vi "Create Test Report from Template.vi"() -> ()   [LabVIEW 2013]
panel:
  in  "Add to Project":u16(ring) items=["<no project selected>", "Caraya.lvproj"]
  in  "Create Test Report Class":bool
  in  "Destination Folder":path
  in  "New Test Report Class Name":string
  # "CARAYA Custom Test Report Class Creator\n\nFill in the destination folder and new TestReport class name."
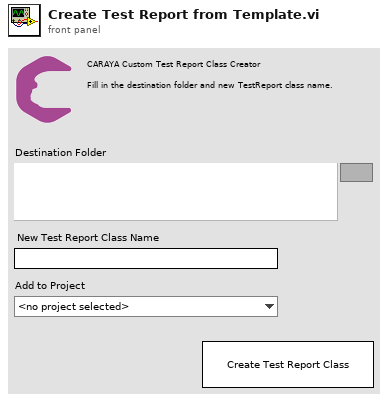
[diagram p1: front panel]
types:
  T1 = enum32{"invalid app kind", "Development System", "Run Time System", "Student Edition", "Embedded LabVIEW", "Evaluation", "Custom"}
  T2 = enum8{"Enabled", "Disabled", "Disabled and Grayed Out"}
  T3 = enum32{"Invalid", "Standard", "Closed", "Hidden", "Minimized", "Maximized"}
  T4 = cluster{"Core":cluster{"Current VI Reference":refnum<vi>, "Close Panel on Exit?":bool}, "ClassName":string, "Path":path, "auto-path":bool, "Menu Launch AppRef":refnum<vi>, "Projects[]":refnum<vi>[], "NewClassPath":path}
  T5 = cluster{"Current VI Reference":refnum<vi>, "Close Panel on Exit?":bool}
  T6 = enum32{"Invalid", "Standard", "Closed", "Hidden", "Minimized", "Maximized"}[]
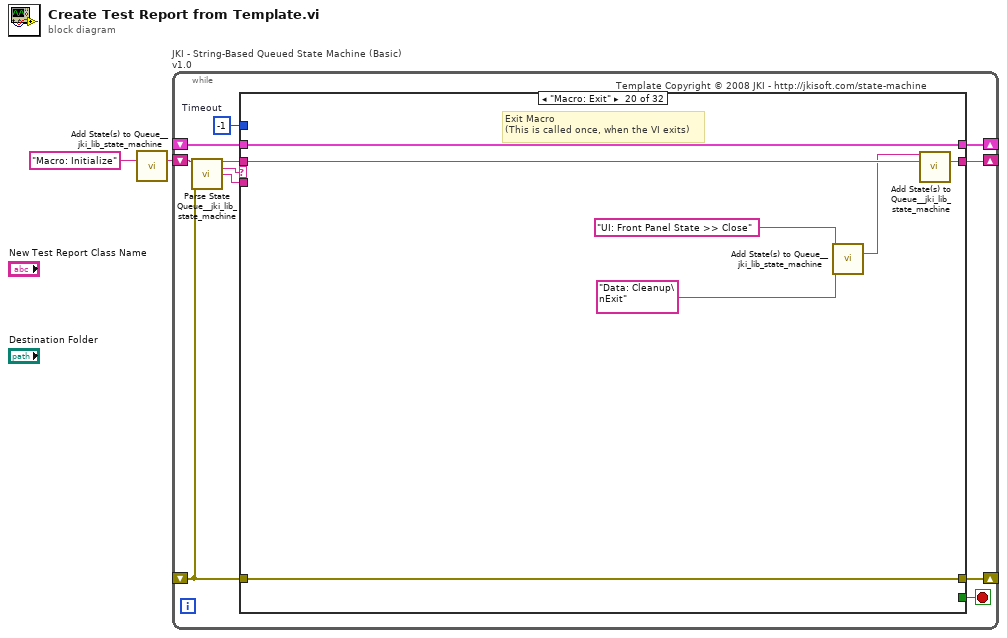
[diagram p0: block diagram]
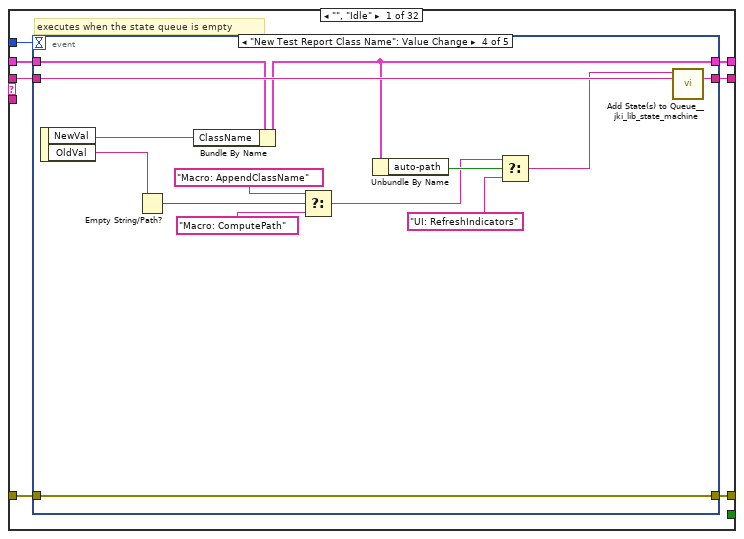
[diagram p2: hidden frame]
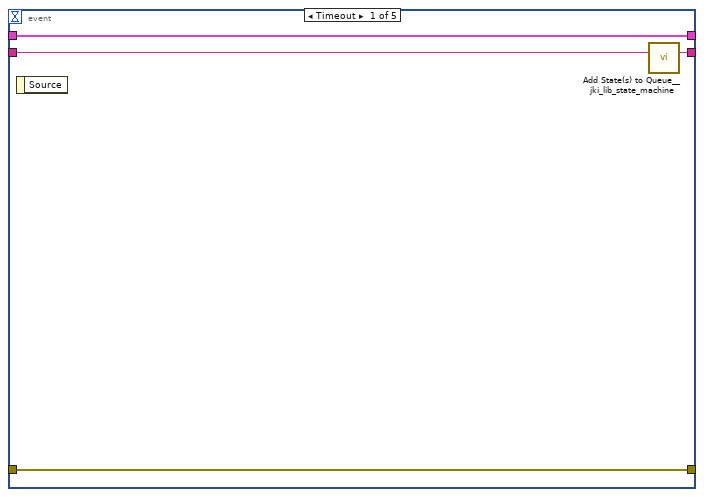
[diagram p3: hidden frame]
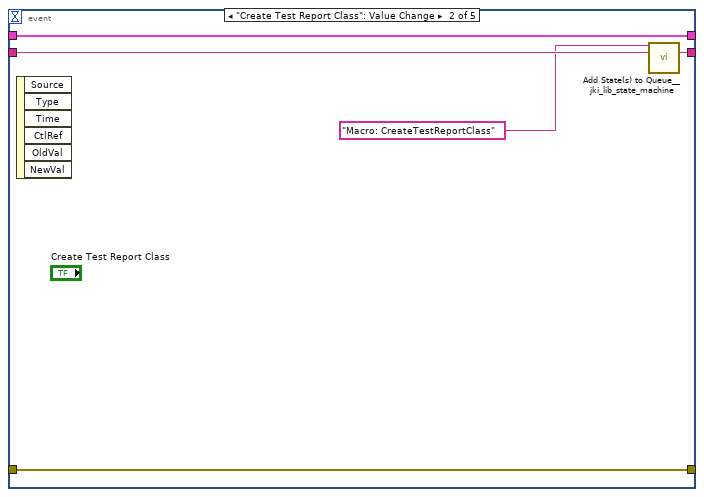
[diagram p4: hidden frame]
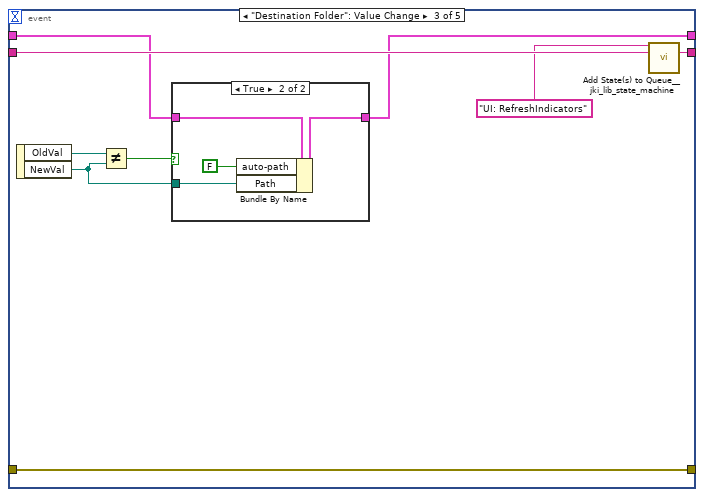
[diagram p5: hidden frame]
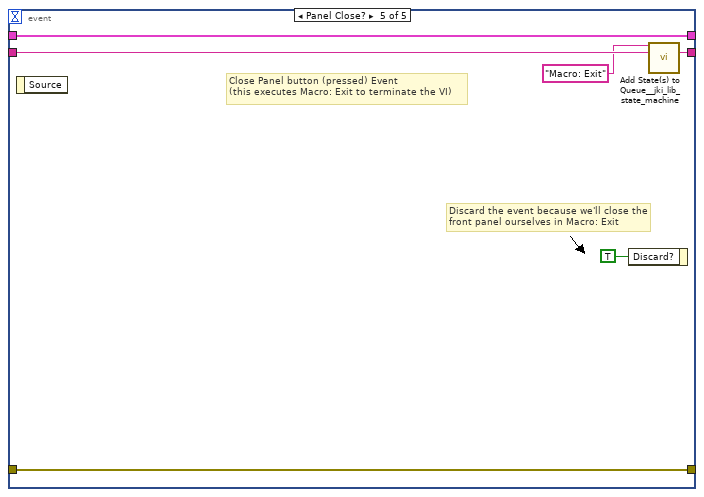
[diagram p7: hidden frame]
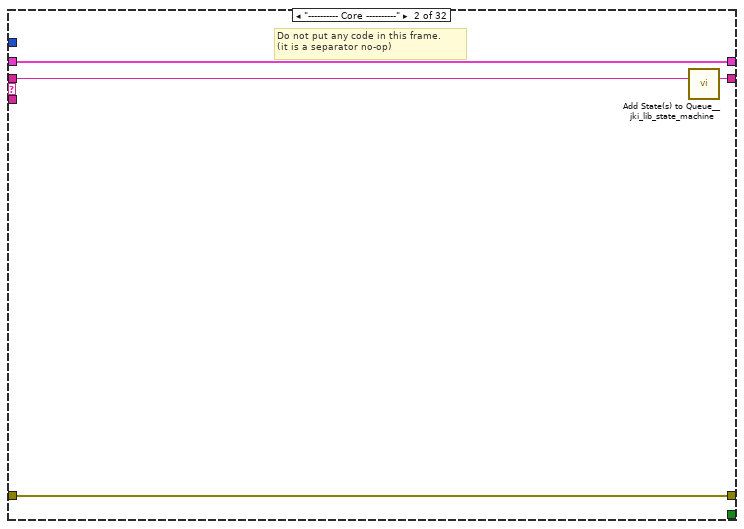
[diagram p8: hidden frame]
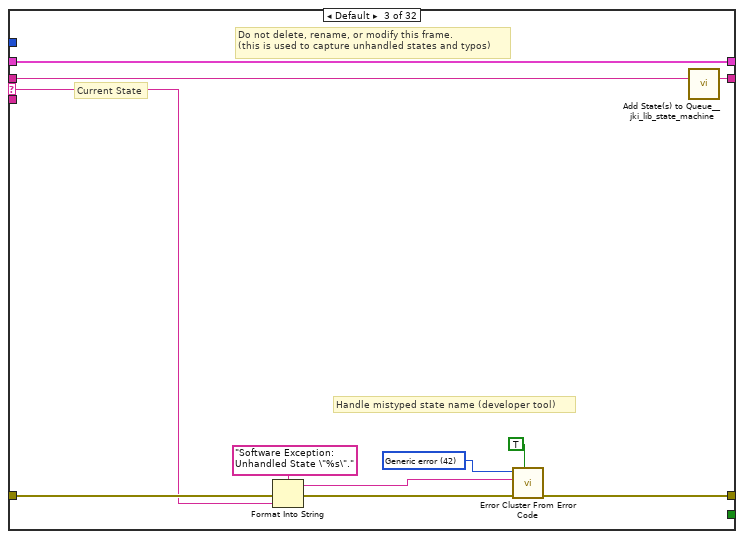
[diagram p9: hidden frame]
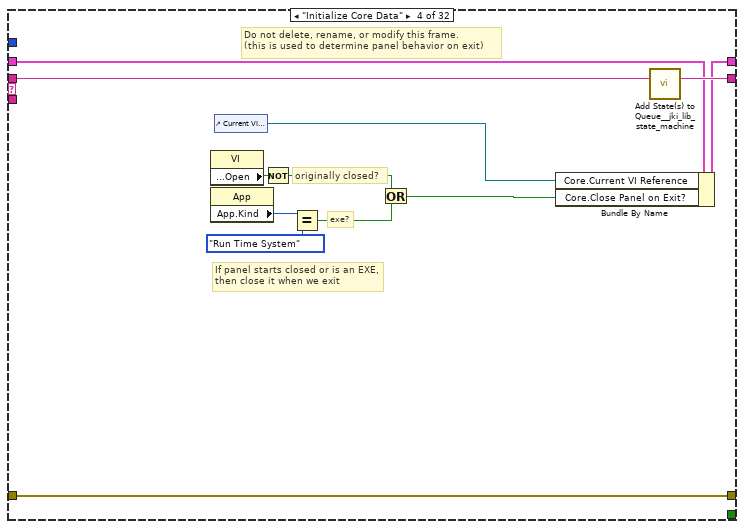
[diagram p10: hidden frame]
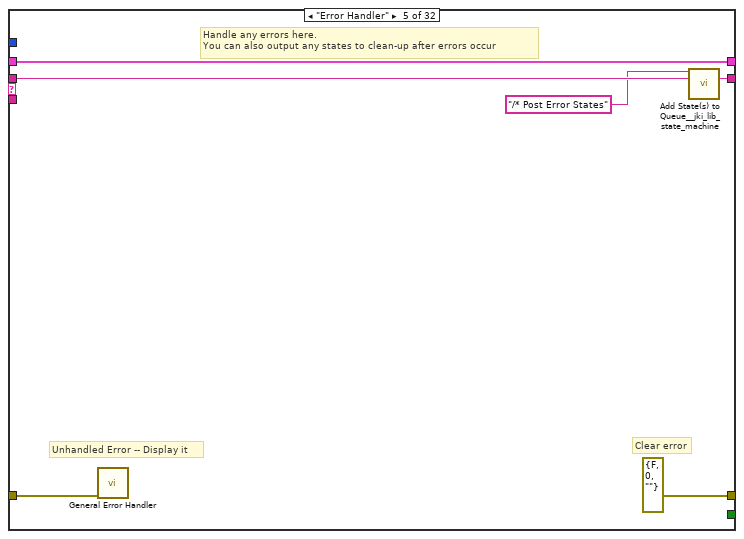
[diagram p11: hidden frame]
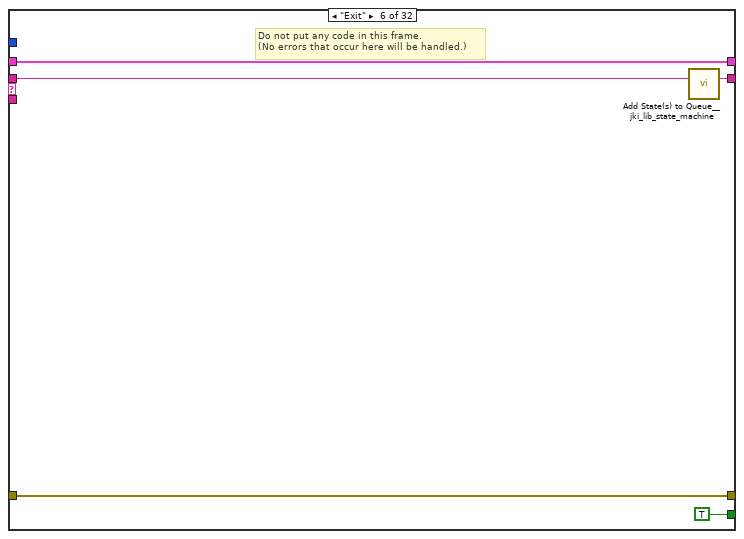
[diagram p12: hidden frame]
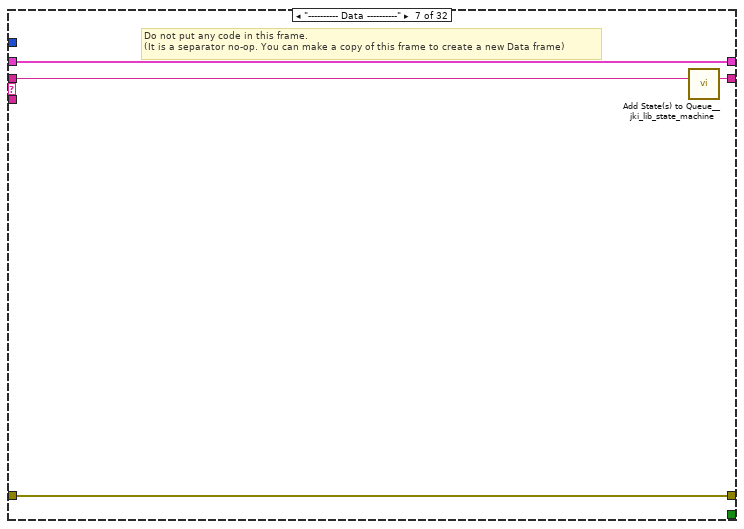
[diagram p13: hidden frame]
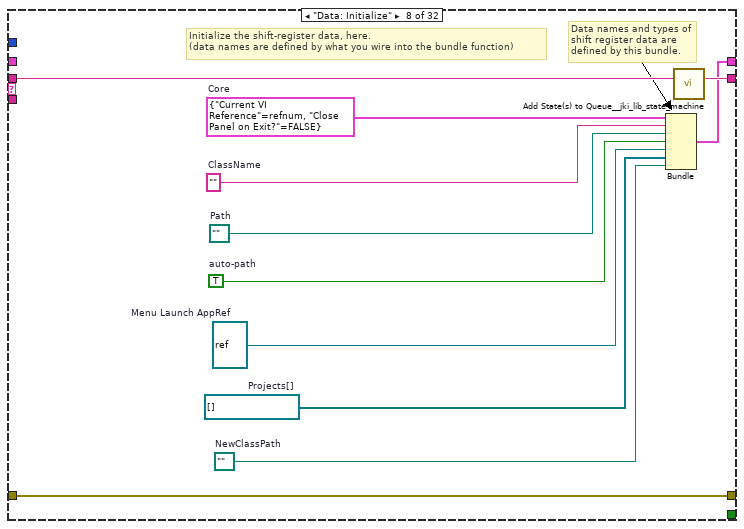
[diagram p14: hidden frame]
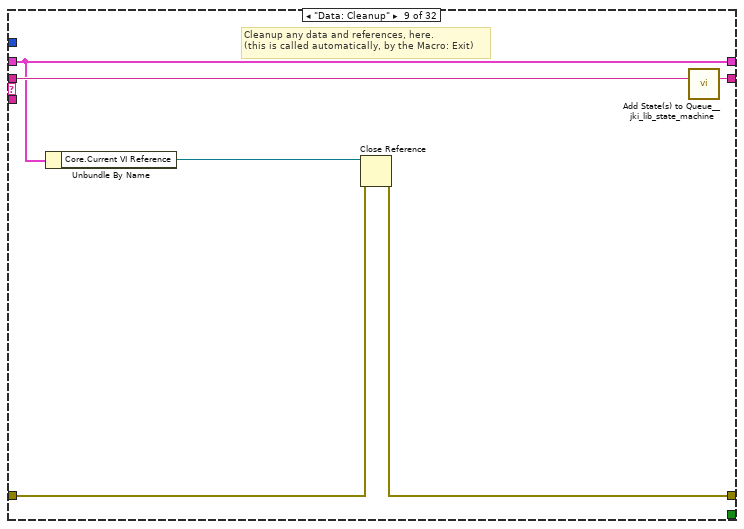
[diagram p15: hidden frame]
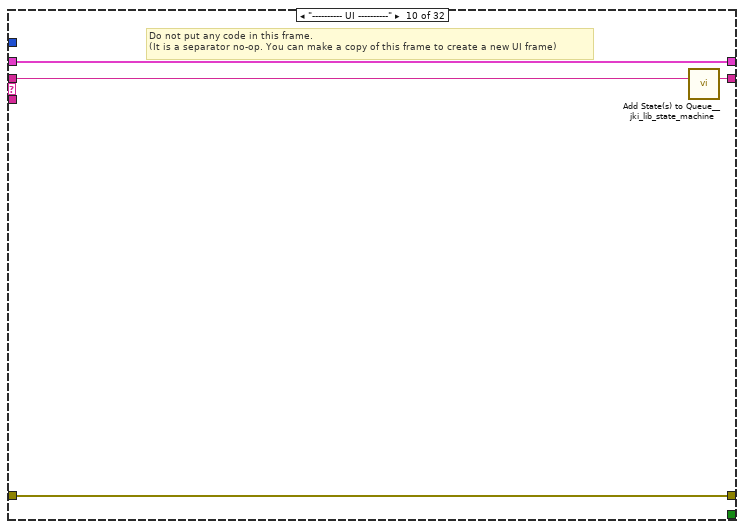
[diagram p16: hidden frame]
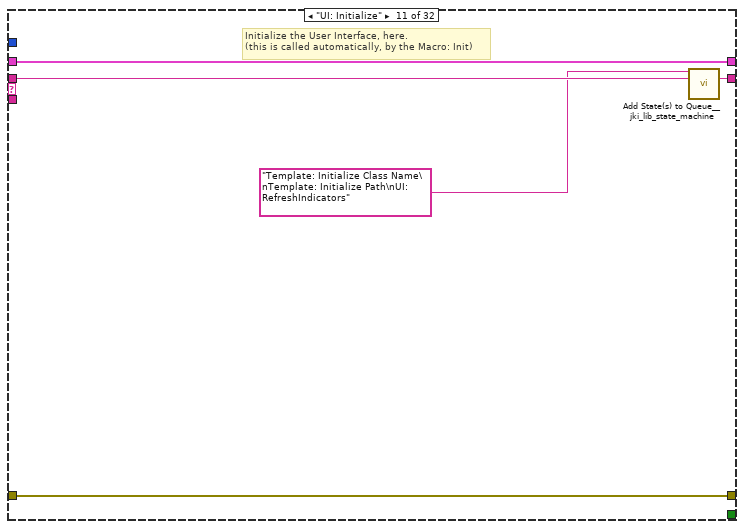
[diagram p17: hidden frame]
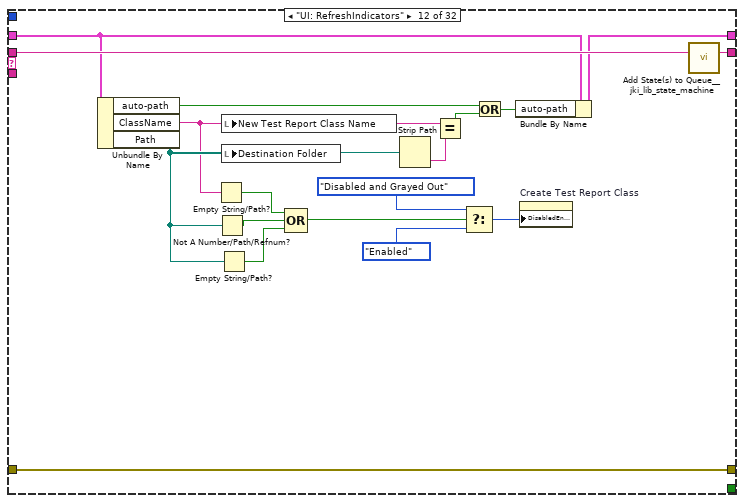
[diagram p18: hidden frame]
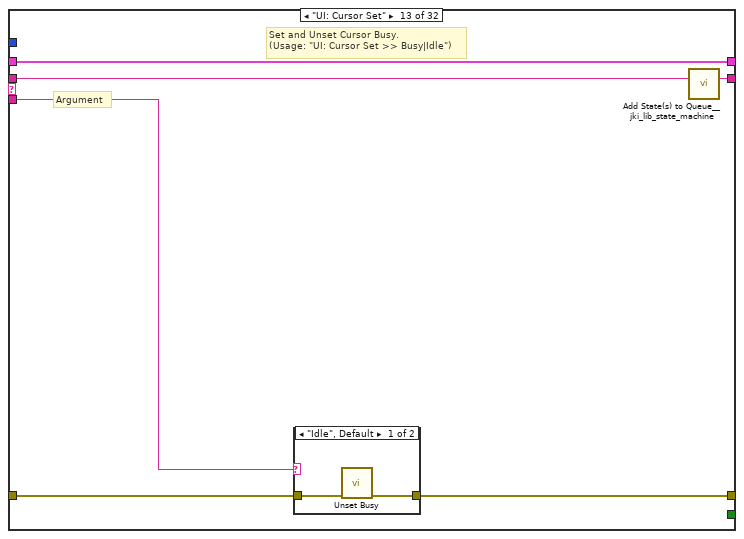
[diagram p19: hidden frame]
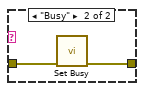
[diagram p20: hidden frame]
diagram:
  n1 = call <vilib>:"Add State(s) to Queue__jki_lib_state_machine.vi"("State(s) in (\"\")"="Macro: Initialize") -> ("States Out"=w2:string)  [unwired: 14 in]
  n2 = while "JKI - String-Based Queued State Machine (Basic) v1.0" {
    shift-right: [w6] -> _
    shift-left: _ -> [w5]
    shift-right: [w9] -> _
    shift-left: _ -> [w3]
    shift-right: [w8] -> _
    shift-left: w2 -> [w10]
    stop <- w7 stop-if-true
    w4 = -1  # Timeout
    # "Template Copyright © 2008 JKI - http://jkisoft.com/state-machine"
    n3 = call <vilib>:"Parse State Queue__jki_lib_state_machine.vi"("State Queue"=w10, "Error In (no error)"=w3) -> ("Remaining States"=w12:string, "Current State"=w13:string, "Arguments"=w11:string)  [unwired: 11 in]
    n4 = case shown="\"Macro: Exit\"" w13 {
      selector: w13 -> [_ _ w68 _ _ _ _ _ _ _ _ _ _ _ _ _ _ _ _ _ _ _ _ _ _ _ _ _ _ _ _ _]
      tunnel: w12 -> [w20 w67 w72 w90 w96 w101 w105 w116 w122 w126 w131 w149 w155 w166 w192 w197 w202 w207 w212 w219 w223 w238 w246 w254 w270 w299 w320 w349 w359 w369 w379 w389]
      tunnel: w11 -> [_ _ _ _ _ _ _ _ _ _ _ _ w150 w160 _ _ _ _ _ _ _ _ _ _ _ _ _ _ _ _ _ _]
      tunnel: w5 -> [w18 w64 w70 w81 w93 w99 w102 _ w117 w123 w128 w136 w153 w162 w189 w194 w199 w204 w209 w216 w220 w236 w243 w248 w259 w295 w316 w345 w354 w364 w374 w387]
      tunnel: [w17 w65 w74 w87 errorcluster {"status"=FALSE, "code"=0, "source"=""} ("error out") w98 w103 w113 w118 w124 w129 w147 w151 w163 w190 w195 w200 w205 w210 w217 w221 w224 w244 w252 w268 w297 w318 w332 w350 w360 w370 w380] -> w9
      tunnel: w3 -> [w16 w65 w73 w87 w92 w98 w103 w113 w119 w124 w129 w147 w152 w164 w190 w195 w200 w205 w210 w217 w221 w225 w244 w252 w268 w297 w318 w335 w356 w366 w376 w381]
      tunnel: [w19 w66 w71 w89 w95 w100 w104 w115 w121 w125 w130 w148 w154 w165 w191 w196 w201 w206 w211 w218 w222 w237 w245 w253 w269 w298 w319 w348 w358 w368 w378 w388] -> w8
      tunnel: [_ _ _ _ _ TRUE _ _ _ _ _ _ _ _ _ _ _ _ _ _ _ _ _ _ _ _ _ _ _ _ _ _] -> w7
      tunnel: [w15 w64 w70 w88 w93 w99 w102 w114 w117 w123 w128 w135 w153 w162 w189 w194 w199 w204 w209 w216 w220 w235 w243 w247 w267 w296 w317 w344 w354 w364 w374 w387] -> w6
      tunnel: w4 -> [w14 _ _ _ _ _ _ _ _ _ _ _ _ _ _ _ _ _ _ _ _ _ _ _ _ _ _ _ _ _ _ _]
      frame "", "Idle" {
        # "executes when the state queue is empty"
        n5 = event shown="[3] \"New Test Report Class Name\": Value Change" {
          selector: _ -> [_ _ _ _ _]
          dyn-events: _ -> [_ _ _ _ _]
          timeout: w14 -> [_ _ _ _ _]
          tunnel: w20 -> [w24 w29 w38 w57 w63]
          tunnel: [w23 w28 w37 w56 w62] -> w19
          tunnel: w18 -> [w21 w26 w34 w54 w60]
          tunnel: [w22 w27 w36 w55 w61] -> w17
          tunnel: w16 -> [w22 w27 w36 w55 w61]
          tunnel: [w21 w26 w31 w53 w60] -> w15
          event Timeout {
            n6 = event-data() -> ()  [unwired: 1 in, 1 out]
            n7 = call <vilib>:"Add State(s) to Queue__jki_lib_state_machine.vi"("State(s) in (\"\")"=w24) -> ("States Out"=w23:string)  [unwired: 14 in]
          }
          event "Create Test Report Class": Value Change {
            n8 = event-data() -> ()  [unwired: 1 in, 6 out]
            n9 = call <vilib>:"Add State(s) to Queue__jki_lib_state_machine.vi"("State(s) in Front (\"\")"="Macro: CreateTestReportClass", "State(s) in (\"\")"=w29) -> ("States Out"=w28:string)  [unwired: 13 in]
          }
          event "Destination Folder": Value Change {
            n10 = event-data() -> ("OldVal"=w35:path, "NewVal"=w32:path)  [unwired: 1 in]
            n11 = Not Equal?(x=w35, y=w32) -> (x != y?=w33:bool)
            n12 = case shown="True" w33 {
              tunnel: [w39 w43] -> w31
              tunnel: w34 -> [w39 w42]
              tunnel: w32 -> [_ w41]
              frame False {
              }
              frame True {
                n13 = Bundle By Name(cluster=w42, "auto-path"=FALSE, "Path"=w41) -> (w43:T4)
              }
            }
            n14 = call <vilib>:"Add State(s) to Queue__jki_lib_state_machine.vi"("State(s) in Front (\"\")"="UI: RefreshIndicators", "State(s) in (\"\")"=w38) -> ("States Out"=w37:string)  [unwired: 13 in]
          }
          event "New Test Report Class Name": Value Change {
            n15 = event-data() -> ("NewVal"=w52:string, "OldVal"=w49:string)  [unwired: 1 in]
            n16 = Empty String/Path?(string/path=w49) -> (empty?=w48:bool)
            n17 = Bundle By Name(cluster=w54, "ClassName"=w52) -> (w53:T4)
            n18 = Select(t="Macro: AppendClassName", s=w48, f="Macro: ComputePath") -> (s? t:f=w45:string)
            n19 = Unbundle By Name(w53) -> ("auto-path"=w51:bool)
            n20 = Select(t=w45, s=w51, f="UI: RefreshIndicators") -> (s? t:f=w50:string)
            n21 = call <vilib>:"Add State(s) to Queue__jki_lib_state_machine.vi"("State(s) in Front (\"\")"=w50, "State(s) in (\"\")"=w57) -> ("States Out"=w56:string)  [unwired: 13 in]
          }
          event Panel Close? {
            # "Discard the event because we'll close the front panel ourselves in Macro: Exit"
            # "Close Panel button (pressed) Event\n(this executes Macro: Exit to terminate the VI)"
            n22 = event-data() -> ()  [unwired: 1 in, 1 out]
            n23 = event-data("Discard?"=TRUE) -> ()  [unwired: 1 in, 1 out]
            n24 = call <vilib>:"Add State(s) to Queue__jki_lib_state_machine.vi"("State(s) in Front (\"\")"="Macro: Exit", "State(s) in (\"\")"=w63) -> ("States Out"=w62:string)  [unwired: 13 in]
          }
        }
      }
      frame "---------- Core ----------" {
        # "Do not put any code in this frame.\n(it is a separator no-op)"
        n25 = call <vilib>:"Add State(s) to Queue__jki_lib_state_machine.vi"("State(s) in (\"\")"=w67) -> ("States Out"=w66:string)  [unwired: 14 in]
      }
      frame Default {
        w77 = 42 items=["No error", "Argument error", "Memory is full", "Out of zone", "End of file", "File already open", "Generic file I/O error", "File not found", "File permission error", "Disk is full", "Duplicate path", "Too many files open", "System feature not enabled", "Resource file not found", "Cannot add resource", "Resource not found", "Image not found", "Image memory error", "Pen does not exist", "Config type invalid", "Config token not found", "Config parse error", "Config memory error", "Bad external code format", "Bad external code offset", "External code not present", "Null window", "Destroy window error", "Null menu", "Print aborted", "Bad print record", "Print driver error", "Windows error during printing", "Memory error during printing", "Print dialog error", "Generic print error", "Invalid device refnum", "Device not found", "Device parameter error", "Device unit error", "Cannot open device", "Device call aborted", "Generic error", "Cancelled by user", "Object ID too low", "Object ID too high", "Object not in heap", "Unknown heap", "Unknown object (invalid DefProc)", "Unknown object (DefProc not in table)", "Message out of range", "Invalid (null) method", "Unknown message", "Manager call not supported", "Bad address", "Network operation in progress", "Network operation timed out", "Connection is busy", "Network attribute not supported", "Network error", "Address in use", "System out of memory", "Connection aborted", "Connection refused", "Not connected", "Already connected", "Connection closed", "Initialization error (interapplication manager)", "Bad occurrence", "Wait on unbound occurrence handler", "Occurrence queue overflow", "Datalog type conflict", "Unused", "Unrecognized type (interapplication manager)", "Memory corrupt", "Failed to make temporary DLL", "Old CIN version", "Drag socket not found", "Failed to load drop-object", "Failed to register OLE object", "Failed to release OLE object", "Format specifier type mismatch", "Unknown format specifier", "Too few format specifiers", "Too many format specifiers", "Scan failed", "Newer CIN version", "Error converting to variant", "Runtime menu error", "Password tampered", "Variant attribute not found", "Incompatible variant data type", "Event data is not available", "Event Store is not present", "Occurrence is not found", "Event Queue is not created", "Event info is not available", "Refnum passed is NULL", "Error retrieving Class GUID", "Error retrieving CoClass GUID", "Error retrieving TypeLib GUID.", "Bad built application magic bytes.", "Specific driver is different from the specific driver associated with the Logical Name.", "There is no session opened to the class driver.", "Max Error", "MAX - Error with config objects", "MAX - Error loading configuration", "MAX - Group not supported"]
        # "Current State"
        # "Do not delete, rename, or modify this frame.\n(this is used to capture unhandled states and typos)"
        # "Handle mistyped state name (developer tool)"
        n26 = Format Into String(format string="Software Exception: Unhandled State \"%s\"." ("message"), error in=w73, w68) -> (resulting string=w76:string, error out=w75:errorcluster)  [unwired: 1 in]
        n27 = call <vilib>:"Error Cluster From Error Code.vi"("show call chain? (False)"=TRUE, "error in (no error)"=w75, "error message (\"\")"=w76, "error code (0)"=w77) -> ("error out"=w74:errorcluster)  [unwired: 5 in]
        n28 = call <vilib>:"Add State(s) to Queue__jki_lib_state_machine.vi"("State(s) in (\"\")"=w72) -> ("States Out"=w71:string)  [unwired: 14 in]
      }
      frame "Initialize Core Data" {
        # "Do not delete, rename, or modify this frame.\n(this is used to determine panel behavior on exit)"
        # "originally closed?"
        # "exe?"
        # "If panel starts closed or is an EXE, then close it when we exit"
        n29 = property class="VI"() -> ("Front Panel.Open"=w86:bool)  [unwired: 2 in, 2 out]
        n30 = property class="App"() -> ("App.Kind"=w85:T1)  [unwired: 2 in, 2 out]
        n31 = control-ref of="Current VI Reference"() -> (w79:refnum<vi>)
        n32 = Not(x=w86) -> (.not. x?=w83:bool)
        n33 = Equal?(x=w85, y=T1."Run Time System" ("Application:Kind")) -> (x = y?=w82:bool)
        n34 = Or(x=w83, y=w82) -> (x .or. y?=w80:bool)
        n35 = Bundle By Name(cluster=w81, "Core.Current VI Reference"=w79, "Core.Close Panel on Exit?"=w80) -> (w88:T4)
        n36 = call <vilib>:"Add State(s) to Queue__jki_lib_state_machine.vi"("State(s) in (\"\")"=w90) -> ("States Out"=w89:string)  [unwired: 14 in]
      }
      frame "Error Handler" {
        # "Unhandled Error -- Display it"
        # "Handle any errors here.\nYou can also output any states to clean-up after errors occur"
        # "Clear error"
        n37 = call <vilib>:"General Error Handler.vi"("error in (no error)"=w92) -> ()  [unwired: 10 in, 5 out]
        n38 = call <vilib>:"Add State(s) to Queue__jki_lib_state_machine.vi"("State(s) in Front (\"\")"="/* Post Error States", "State(s) in (\"\")"=w96) -> ("States Out"=w95:string)  [unwired: 13 in]
      }
      frame "Exit" {
        # "Do not put any code in this frame.\n(No errors that occur here will be handled.)"
        n39 = call <vilib>:"Add State(s) to Queue__jki_lib_state_machine.vi"("State(s) in (\"\")"=w101) -> ("States Out"=w100:string)  [unwired: 14 in]
      }
      frame "---------- Data ----------" {
        # "Do not put any code in this frame.\n(It is a separator no-op. You can make a copy of this frame to create a new Data frame)"
        n40 = call <vilib>:"Add State(s) to Queue__jki_lib_state_machine.vi"("State(s) in (\"\")"=w105) -> ("States Out"=w104:string)  [unwired: 14 in]
      }
      frame "Data: Initialize" {
        w106 = path ""  # NewClassPath
        w107 = refnum<vi>[] []  # Projects[]
        w108 = refnum<vi> refnum  # Menu Launch AppRef
        w109 = TRUE  # auto-path
        w110 = path ""  # Path
        w111 = T5 {"Current VI Reference"=refnum, "Close Panel on Exit?"=FALSE}  # Core
        w112 = ""  # ClassName
        # "Data names and types of shift register data are defined by this bundle."
        # "Initialize the shift-register data, here.\n(data names are defined by what you wire into the bundle function)"
        n41 = Bundle("Core"=w111, "ClassName"=w112, "Path"=w110, "auto-path"=w109, "Menu Launch AppRef"=w108, "Projects[]"=w107, "NewClassPath"=w106) -> (w114:T4)  [unwired: 1 in]
        n42 = call <vilib>:"Add State(s) to Queue__jki_lib_state_machine.vi"("State(s) in (\"\")"=w116) -> ("States Out"=w115:string)  [unwired: 14 in]
      }
      frame "Data: Cleanup" {
        # "Cleanup any data and references, here.\n(this is called automatically, by the Macro: Exit)"
        n43 = Unbundle By Name(w117) -> ("Core.Current VI Reference"=w120:refnum<vi>)
        n44 = Close Reference(reference=w120, error in (no error)=w119) -> (error out=w118:errorcluster)
        n45 = call <vilib>:"Add State(s) to Queue__jki_lib_state_machine.vi"("State(s) in (\"\")"=w122) -> ("States Out"=w121:string)  [unwired: 14 in]
      }
      frame "---------- UI ----------" {
        # "Do not put any code in this frame.\n(It is a separator no-op. You can make a copy of this frame to create a new UI frame)"
        n46 = call <vilib>:"Add State(s) to Queue__jki_lib_state_machine.vi"("State(s) in (\"\")"=w126) -> ("States Out"=w125:string)  [unwired: 14 in]
      }
      frame "UI: Initialize" {
        # "Initialize the User Interface, here.\n(this is called automatically, by the Macro: Init)"
        n47 = call <vilib>:"Add State(s) to Queue__jki_lib_state_machine.vi"("State(s) in Front (\"\")"="Template: Initialize Class Name\nTemplate: Initialize Path\nUI: RefreshIndicators" ("Text.Text"), "State(s) in (\"\")"=w131) -> ("States Out"=w130:string)  [unwired: 13 in]
      }
      frame "UI: RefreshIndicators" {
        n48 = Unbundle By Name(w136) -> ("auto-path"=w134:bool, "ClassName"=w137:string, "Path"=w139:path)
        n49 = Empty String/Path?(string/path=w137) -> (empty?=w146:bool)
        n50 = Not A Number/Path/Refnum?(number/path/refnum=w139) -> (NaN/Path/Refnum?=w145:bool)
        n51 = Empty String/Path?(string/path=w139) -> (empty?=w144:bool)
        n52 = local write "New Test Report Class Name"(w137) -> ()
        n53 = local write "Destination Folder"(w139) -> ()
        n54 = Compound Arithmetic op=OR(w146, w145, w144) -> (w142:bool)
        n55 = Strip Path(path=w139) -> (name=w138:string)  [unwired: 1 out]
        n56 = Equal?(x=w137, y=w138) -> (x = y?=w133:bool)
        n57 = Select(t=T2."Disabled and Grayed Out" ("Disabled"), s=w142, f=T2."Enabled" ("Disabled")) -> (s? t:f=w140:T2)
        n58 = Or(x=w134, y=w133) -> (x .or. y?=w132:bool)
        n59 = Bundle By Name(cluster=w136, "auto-path"=w132) -> (w135:T4)
        n60 = property on="Create Test Report Class" class="Bool"("DisabledEnum"=w140) -> ()  [unwired: 2 in, 2 out]
        n61 = call <vilib>:"Add State(s) to Queue__jki_lib_state_machine.vi"("State(s) in (\"\")"=w149) -> ("States Out"=w148:string)  [unwired: 14 in]
      }
      frame "UI: Cursor Set" {
        # "Argument"
        # "Set and Unset Cursor Busy.\n(Usage: \"UI: Cursor Set >> Busy|Idle\")"
        n62 = case shown="\"Idle\", Default" w150 {
          tunnel: w152 -> [w157 w159]
          tunnel: [w156 w158] -> w151
          frame "Idle", Default {
            n63 = call <vilib>:"Unset Busy.vi"("error in (no error)"=w157) -> ("error out"=w156:errorcluster)  [unwired: 10 in]
          }
          frame "Busy" {
            n64 = call <vilib>:"Set Busy.vi"("error in (no error)"=w159) -> ("error out"=w158:errorcluster)  [unwired: 9 in, 1 out]
          }
        }
        n65 = call <vilib>:"Add State(s) to Queue__jki_lib_state_machine.vi"("State(s) in (\"\")"=w155) -> ("States Out"=w154:string)  [unwired: 14 in]
      }
      frame "UI: Front Panel State" {
        # "Argument"
        # "Set Front Panel Open or Closed\n(Usage: \"UI: Front Panel State >> Open|Close\")"
        n66 = Unbundle By Name(w162) -> ("Core.Current VI Reference"=w161:refnum<vi>)
        n67 = case shown="\"Open\", Default" w160 {
          tunnel: w164 -> [w170 w183]
          tunnel: [w172 w184] -> w163
          tunnel: w161 -> [w171 w181]
          frame "Open", Default {
            n68 = property class="VI"(reference=w171, error in=w170) -> (reference out=w168:refnum<vi>, error out=w169:errorcluster, "Front Panel.Open"=w167:bool)
            n69 = case shown="False" w167 {
              tunnel: [w175 w178] -> w172
              tunnel: w169 -> [w174 w178]
              tunnel: w168 -> [w173 _]
              frame False {
                n70 = invoke class="VI" method="FP.Open"(reference=w173, error in=w174, "Activate"=TRUE, "State"=T3."Standard") -> (error out=w175:errorcluster)  [unwired: 1 in, 4 out]
              }
              frame True {
              }
            }
          }
          frame "Close" {
            n71 = property class="VI"(reference=w181, error in=w183) -> (reference out=w180:refnum<vi>, error out=w182:errorcluster, "Front Panel.Open"=w179:bool)
            n72 = case shown="True" w179 {
              tunnel: [w185 w188] -> w184
              tunnel: w182 -> [w185 w187]
              tunnel: w180 -> [_ w186]
              frame False {
              }
              frame True {
                n73 = invoke class="VI" method="FP.Close"(reference=w186, error in=w187) -> (error out=w188:errorcluster)  [unwired: 1 in, 2 out]
              }
            }
          }
        }
        n74 = call <vilib>:"Add State(s) to Queue__jki_lib_state_machine.vi"("State(s) in (\"\")"=w166) -> ("States Out"=w165:string)  [unwired: 14 in]
      }
      frame "---------- Macro ----------" {
        # "Do not put any code in this frame.\n(It is a separator no-op. You can make a copy of this frame to create a new Macro frame)"
        n75 = call <vilib>:"Add State(s) to Queue__jki_lib_state_machine.vi"("State(s) in (\"\")"=w192) -> ("States Out"=w191:string)  [unwired: 14 in]
      }
      frame "Macro: Initialize" {
        w193 = "Data: Initialize\nInitialize Core Data\nProject: Initialize\nUI: Initialize\nUI: Front Panel State >> Open\n\n"  # Data: Initialize Initialize Core Data Project: Initialize UI: Initialize UI: Front Panel State >> Open
        # "Initialization Macro\n(This is called once, when the VI starts)"
        n76 = call <vilib>:"Add State(s) to Queue__jki_lib_state_machine.vi"("State(s) in Front (\"\")"=w193, "State(s) in (\"\")"=w197) -> ("States Out"=w196:string)  [unwired: 13 in]
      }
      frame "Macro: ComputePath" {
        n77 = call <vilib>:"Add State(s) to Queue__jki_lib_state_machine.vi"("State(s) in Front (\"\")"="Template: Adjust Path from ClassName\nUI: RefreshIndicators", "State(s) in (\"\")"=w202) -> ("States Out"=w201:string)  [unwired: 13 in]
      }
      frame "Macro: AppendClassName" {
        n78 = call <vilib>:"Add State(s) to Queue__jki_lib_state_machine.vi"("State(s) in Front (\"\")"="Template: Append ClassName to Path\nUI: RefreshIndicators", "State(s) in (\"\")"=w207) -> ("States Out"=w206:string)  [unwired: 13 in]
      }
      frame "Macro: CreateTestReportClass" {
        n79 = call <vilib>:"Add State(s) to Queue__jki_lib_state_machine.vi"("State(s) in Front (\"\")"="Template: Create TestReport\nTemplate: Rename Operands\nTemplate: Change VI Names\nTemplate: Update Icon\nTemplate: Post-Action", "State(s) in (\"\")"=w212) -> ("States Out"=w211:string)  [unwired: 13 in]
      }
      frame "Macro: Exit" {
        # "Exit Macro\n(This is called once, when the VI exits)"
        n80 = call <vilib>:"Add State(s) to Queue__jki_lib_state_machine.vi"("State(s) in Front (\"\")"="UI: Front Panel State >> Close", "State(s) at Back (\"\")"="Data: Cleanup\nExit") -> ("States Out"=w214:string)  [unwired: 13 in]
        n81 = call <vilib>:"Add State(s) to Queue__jki_lib_state_machine.vi"("State(s) in Front (\"\")"=w214, "State(s) in (\"\")"=w219) -> ("States Out"=w218:string)  [unwired: 13 in]
      }
      frame "---------- Project ----------" {
        n82 = call <vilib>:"Add State(s) to Queue__jki_lib_state_machine.vi"("State(s) in (\"\")"=w223) -> ("States Out"=w222:string)  [unwired: 14 in]
      }
      frame "Project: Initialize" {
        # "List projects in\nthis AppInstance"
        # "Figure out from which AppInstance the call was made"
        n83 = property class="App"() -> (reference out=w234:refnum<vi>, error out=w232:errorcluster, "App.MenuLaunchApp"=w233:refnum<vi>)  [unwired: 2 in]
        n84 = Select(t=w234, s=w232, f=w233) -> (s? t:f=w227:refnum<vi>)
        n85 = property class="App"(reference=w227, error in=w225) -> (error out=w228:errorcluster, "Project"=w226:refnum<vi>[])  [unwired: 1 out]
        n86 = for {
          tunnel: w226 -> [w242] mode=indexing
          tunnel: [w241] -> w229 mode=indexing
          shift-right: [w239] -> w224
          shift-left: w228 -> [w240]
          n87 = property class="Project"(reference=w242, error in=w240) -> (error out=w239:errorcluster, "Name"=w241:string)  [unwired: 1 out]
        }
        n88 = Bundle By Name(cluster=w236, "Projects[]"=w226) -> (w235:T4)
        n89 = Build Array (concatenate)("<no project selected>", w229) -> (w230:string[])
        n90 = property on="Add to Project" class="Ring (strict)"("Strings []"=w230) -> ()  [unwired: 2 in, 2 out]
        n91 = call <vilib>:"Add State(s) to Queue__jki_lib_state_machine.vi"("State(s) in (\"\")"=w238) -> ("States Out"=w237:string)  [unwired: 14 in]
      }
      frame "---------- Template ----------" {
        n92 = call <vilib>:"Add State(s) to Queue__jki_lib_state_machine.vi"("State(s) in (\"\")"=w246) -> ("States Out"=w245:string)  [unwired: 14 in]
      }
      frame "Template: Initialize Class Name" {
        n93 = property on="New Test Report Class Name" class="Str"() -> ("Text.Text"=w250:string)  [unwired: 2 in, 2 out]
        n94 = Empty String/Path?(string/path=w250) -> (empty?=w251:bool)
        n95 = case shown="True" w251 {
          tunnel: w250 -> [w255 _]
          tunnel: [w255 "myTestReport" ("Text.Text")] -> w249
          frame False {
          }
          frame True {
          }
        }
        n96 = Bundle By Name(cluster=w248, "ClassName"=w249) -> (w247:T4)
        n97 = call <vilib>:"Add State(s) to Queue__jki_lib_state_machine.vi"("State(s) in (\"\")"=w254) -> ("States Out"=w253:string)  [unwired: 14 in]
      }
      frame "Template: Initialize Path" {
        n98 = property on="Destination Folder" class="Path"() -> ("Value"=w262:path)  [unwired: 2 in, 2 out]
        n99 = Unbundle By Name(w259) -> ("ClassName"=w258:string)
        n100 = Unbundle By Name(w259) -> ("Projects[]"=w260:refnum<vi>[])
        n101 = Not A Number/Path/Refnum?(number/path/refnum=w262) -> (NaN/Path/Refnum?=w261:bool)
        n102 = Empty String/Path?(string/path=w262) -> (empty?=w264:bool)
        n103 = Or(x=w261, y=w264) -> (x .or. y?=w263:bool)
        n104 = case shown="True" w263 {
          tunnel: w262 -> [w271 _]
          tunnel: [w271 w282] -> w266
          tunnel: w260 -> [_ w281]
          tunnel: w258 -> [_ w277]
          tunnel: [_ w273] -> w257
          frame False {
          }
          frame True {
            n105 = for {
              tunnel: w281 -> [w290] mode=indexing
              tunnel: [w286] -> w276
              tunnel: [w284] -> w280
              tunnel: [w283] -> w275
              i -> [w283]
              stop <- w286 stop-if-true
              w289 = T6 [enum."Standard", enum."Minimized", enum."Maximized"] items=["Invalid", "Standard", "Closed", "Hidden", "Minimized", "Maximized"]
              n106 = property class="Project"(reference=w290) -> ("Path"=w285:path, "Window State"=w288:T3)  [unwired: 1 in, 2 out]
              n107 = Search 1D Array(1D array=w289, element=w288) -> (index of element=w287:i32)  [unwired: 1 in]
              n108 = Strip Path(path=w285) -> (stripped path=w284:path)  [unwired: 1 out]
              n109 = Greater Or Equal To 0?(x=w287) -> (x >= 0?=w286:bool)
            }
            n110 = Increment(x=w275) -> (x+1=w272:i32)
            n111 = call <vilib>:"Application Directory.vi"() -> ("Application Directory"=w279:path)
            n112 = Select(t=w280, s=w276, f=w279) -> (s? t:f=w278:path)
            n113 = Select(t=w272, s=w276, f=0) -> (s? t:f=w273:i32)
            n114 = Build Path(base path=w278, name or relative path=w277) -> (appended path=w282:path)
          }
        }
        n115 = property on="Destination Folder" class="Path"("StartPath"=w266) -> ()  [unwired: 2 in, 2 out]
        n116 = Bundle By Name(cluster=w259, "Path"=w266, "auto-path"=TRUE) -> (w267:T4)
        n117 = property on="Add to Project" class="Ring (strict)"("Value"=w257) -> ()  [unwired: 2 in, 2 out]
        n118 = call <vilib>:"Add State(s) to Queue__jki_lib_state_machine.vi"("State(s) in (\"\")"=w270) -> ("States Out"=w269:string)  [unwired: 14 in]
      }
      frame "Template: Adjust Path from ClassName" {
        n119 = Unbundle By Name(w295) -> ("Path"=w291:path, "ClassName"=w293:string)
        n120 = Empty String/Path?(string/path=w291) -> (empty?=w292:bool)
        n121 = case shown="False" w292 {
          tunnel: w291 -> [w303 _]
          tunnel: [w302 w309] -> w294
          tunnel: w293 -> [w301 w310]
          frame False {
            n122 = Empty String/Path?(string/path=w301) -> (empty?=w300:bool)
            n123 = Strip Path(path=w303) -> (stripped path=w304:path)  [unwired: 1 out]
            n124 = case shown="False" w300 {
              tunnel: w304 -> [w307 w308]
              tunnel: [w306 w308] -> w302
              tunnel: w301 -> [w305 _]
              frame False {
                n125 = Build Path(base path=w307, name or relative path=w305) -> (appended path=w306:path)
              }
              frame True {
              }
            }
          }
          frame True {
            n126 = call <vilib>:"Application Directory.vi"() -> ("Application Directory"=w311:path)
            n127 = Build Path(base path=w311, name or relative path=w310) -> (appended path=w309:path)
          }
        }
        n128 = Bundle By Name(cluster=w295, "Path"=w294) -> (w296:T4)
        n129 = call <vilib>:"Add State(s) to Queue__jki_lib_state_machine.vi"("State(s) in (\"\")"=w299) -> ("States Out"=w298:string)  [unwired: 14 in]
      }
      frame "Template: Append ClassName to Path" {
        n130 = Unbundle By Name(w316) -> ("Path"=w312:path, "ClassName"=w314:string)
        n131 = Empty String/Path?(string/path=w312) -> (empty?=w313:bool)
        n132 = case shown="False" w313 {
          tunnel: w312 -> [w321 _]
          tunnel: [w324 w329] -> w315
          tunnel: w314 -> [w323 w330]
          frame False {
            n133 = Empty String/Path?(string/path=w323) -> (empty?=w322:bool)
            n134 = case shown="False" w322 {
              tunnel: w321 -> [w327 w328]
              tunnel: [w326 w328] -> w324
              tunnel: w323 -> [w325 _]
              frame False {
                n135 = Build Path(base path=w327, name or relative path=w325) -> (appended path=w326:path)
              }
              frame True {
              }
            }
          }
          frame True {
            n136 = call <vilib>:"Application Directory.vi"() -> ("Application Directory"=w331:path)
            n137 = Build Path(base path=w331, name or relative path=w330) -> (appended path=w329:path)
          }
        }
        n138 = Bundle By Name(cluster=w316, "Path"=w315) -> (w317:T4)
        n139 = call <vilib>:"Add State(s) to Queue__jki_lib_state_machine.vi"("State(s) in (\"\")"=w320) -> ("States Out"=w319:string)  [unwired: 14 in]
      }
      frame "Template: Create TestReport" {
        # "For some reason, the MenuLaunch AppRef gets lost.\nUsing the Project App Ref works!"
        n140 = Unbundle By Name(w345) -> ("Projects[]"=w334:refnum<vi>[], "Path"=w347:path, "ClassName"=w346:string)
        n141 = VI Library() -> (path=w343:path)
        n142 = Index Array(array=w334) -> (element=w338:refnum<vi>)  [unwired: 1 in]
        n143 = Build Path(base path=w343, name or relative path=path "addons/_JKI Toolkits/Caraya/classes/Test Report.Template/Test Report.Template.lvclass" ("Path")) -> (appended path=w341:path)
        n144 = property class="Project"(reference=w338, error in=w335) -> (error out=w336:errorcluster, "App Ref"=w337:refnum<vi>)  [unwired: 1 out]
        n145 = invoke class="App" method="LVClass.Open"(reference=w337, error in=w336, "Path"=w341) -> (error out=w339:errorcluster, "LVClass.Open"=w340:refnum<vi>)  [unwired: 1 in, 2 out]
        n146 = invoke class="LVClassLibrary" method="Save a Copy"(reference=w340, error in=w339, "Path"=w347, "New Name"=w346) -> (error out=w332:errorcluster, "New Lib Path"=w333:path)  [unwired: 2 in, 4 out]
        n147 = Bundle By Name(cluster=w345, "NewClassPath"=w333) -> (w344:T4)
        n148 = call <vilib>:"Add State(s) to Queue__jki_lib_state_machine.vi"("State(s) in (\"\")"=w349) -> ("States Out"=w348:string)  [unwired: 14 in]
      }
      frame "Template: Rename Operands" {
        n149 = Unbundle By Name(w354) -> ("Projects[]"=w355:refnum<vi>[], "NewClassPath"=w353:path)
        n150 = Index Array(array=w355) -> (element=w357:refnum<vi>)  [unwired: 1 in]
        n151 = property class="Project"(reference=w357, error in=w356) -> (error out=w351:errorcluster, "App Ref"=w352:refnum<vi>)  [unwired: 1 out]
        n152 = call "_caraya_renameOperands.vi"("error in (no error)"=w351, "Application"=w352, "New Class Path"=w353) -> ("error out"=w350:errorcluster)  [unwired: 8 in]
        n153 = call <vilib>:"Add State(s) to Queue__jki_lib_state_machine.vi"("State(s) in (\"\")"=w359) -> ("States Out"=w358:string)  [unwired: 14 in]
      }
      frame "Template: Change VI Names" {
        n154 = Unbundle By Name(w364) -> ("Projects[]"=w365:refnum<vi>[], "NewClassPath"=w361:path)
        n155 = Index Array(array=w365) -> (element=w367:refnum<vi>)  [unwired: 1 in]
        n156 = property class="Project"(reference=w367, error in=w366) -> (error out=w363:errorcluster, "App Ref"=w362:refnum<vi>)  [unwired: 1 out]
        n157 = call "_caraya_updateVInames.vi"("error in (no error)"=w363, "Application"=w362, "Class Path"=w361) -> ("error out"=w360:errorcluster)  [unwired: 8 in]
        n158 = call <vilib>:"Add State(s) to Queue__jki_lib_state_machine.vi"("State(s) in (\"\")"=w369) -> ("States Out"=w368:string)  [unwired: 14 in]
      }
      frame "Template: Update Icon" {
        n159 = Unbundle By Name(w374) -> ("Projects[]"=w375:refnum<vi>[], "NewClassPath"=w373:path)
        n160 = Index Array(array=w375) -> (element=w377:refnum<vi>)  [unwired: 1 in]
        n161 = property class="Project"(reference=w377, error in=w376) -> (error out=w371:errorcluster, "App Ref"=w372:refnum<vi>)  [unwired: 1 out]
        n162 = call "_caraya_updateLibraryIcon.vi"("error in (no error)"=w371, "Application"=w372, "Class Path"=w373) -> ("error out"=w370:errorcluster)  [unwired: 8 in]
        n163 = call <vilib>:"Add State(s) to Queue__jki_lib_state_machine.vi"("State(s) in (\"\")"=w379) -> ("States Out"=w378:string)  [unwired: 14 in]
      }
      frame "Template: Post-Action" {
        n164 = Unbundle By Name(w387) -> ("NewClassPath"=w382:path, "Projects[]"=w383:refnum<vi>[])
        n165 = To Long Integer(number="Add to Project") -> (32bit integer=w384:i32)
        n166 = Decrement(x=w384) -> (x-1=w385:i32)
        n167 = case shown="Default" w385 {
          selector: w385 -> [w396 _]
          tunnel: w383 -> [w397 _]
          tunnel: w382 -> [w392 _]
          tunnel: w381 -> [w391 w398]
          tunnel: [w390 w398] -> w380
          frame Default {
            n168 = Index Array(array=w397, index=w396) -> (element=w395:refnum<vi>)
            n169 = property class="Project"(reference=w395, error in=w391) -> (error out=w393:errorcluster, "My Computer"=w394:refnum<vi>)  [unwired: 1 out]
            n170 = invoke class="TargetItem" method="AddFile"(reference=w394, error in=w393, "Path"=w392) -> (error out=w390:errorcluster)  [unwired: 1 in, 3 out]
          }
          frame -1 {
          }
        }
        n171 = call <vilib>:"Add State(s) to Queue__jki_lib_state_machine.vi"("State(s) in (\"\")"=w389) -> ("States Out"=w388:string)  [unwired: 14 in]
      }
    }
  }
